vi "BIO_get_fd.vi"(8 "error in (no error)":errorcluster, 11 "BIO in":refnum<class "BIO.lvclass">) -> (0 "error out":errorcluster, 2 "socket fd":i32, 3 "BIO out":refnum<class "BIO.lvclass">)   [LabVIEW 2013, in "OpenSSL Socket.lvlib" / "BIO.lvclass"]
uses:
  BIO.lvclass
  SSL-Lib/SSL-Lib.lvclass/SSL-Lib.ctl
  BIO.lvclass/BIO.ctl
  SSL-Lib/Read Crypto Library Path.vi
  Read Handle.vi
  SSL-Lib/SSL-Lib.lvclass
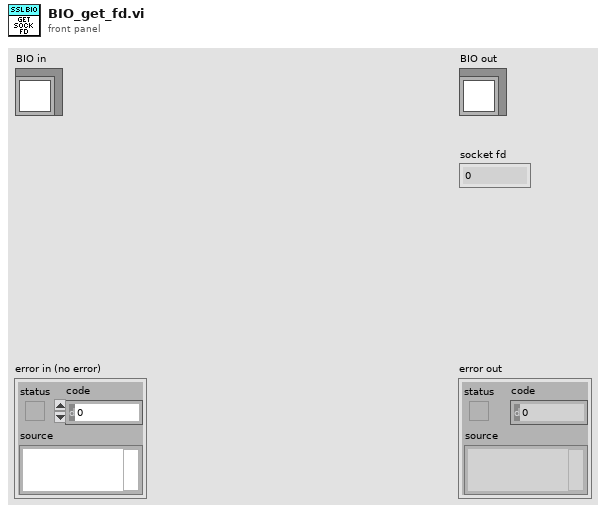
[diagram p1: front panel]
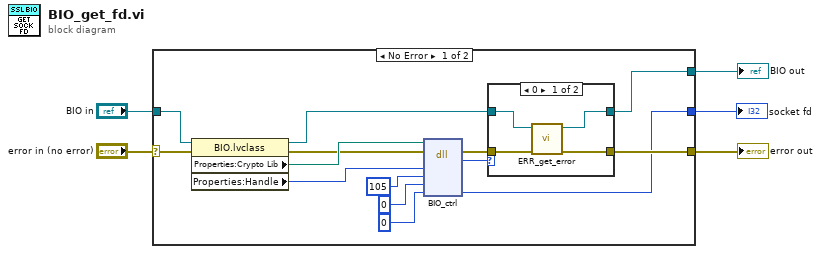
[diagram p0: block diagram]
diagram:
  n1 = case shown="No Error" "error in (no error)" {
    selector: "error in (no error)" -> [w15 w27]
    tunnel: [w7 w27] -> w4
    tunnel: [w8 w26] -> w2
    tunnel: "BIO in" -> [w16 w26]
    tunnel: [w6 _] -> w1
    frame No Error {
      n2 = property class="BIO.lvclass"(reference=w16, error in=w15) -> (reference out=w9:refnum<class "BIO.lvclass">, error out=w12:errorcluster, "Properties:Crypto Lib"=w14:path, "Properties:Handle"=w13:u64)
      n3 = dll-call lib="C:/Program Files (x86)/National Instruments/Shared/nissl/NIlibeay32.dll" fn="BIO_ctrl"(path in=w14, error in=w12, "BIO"=w13, "cmd"=105, "larg"=0, "parg"=0 ("*SSL")) -> (error out=w10:errorcluster, "return type"=w11:i32, "parg"=w6:i32)  [unwired: 4 in, 1 out]
      n4 = case shown="0" w11 {
        tunnel: w10 -> [w23 w25]
        tunnel: [w20 w25] -> w7
        tunnel: w9 -> [w22 w24]
        tunnel: [w21 w24] -> w8
        frame 0 {
          n5 = call "ERR_get_error.vi"("error in (no error)"=w23, "SSL-Lib in"=w22) -> ("error out"=w20:errorcluster, "SSL-Lib out"=w21:refnum<class "BIO.lvclass">)  [unwired: 8 in]
        }
        frame Default {
        }
      }
    }
    frame Error {
    }
  }
  "error out" <- w4
  "BIO out" <- w2
  "socket fd" <- w1
